vi "ex_Get Control Refnum.vi"(8 "error in (no error)":errorcluster, 9 "Name":string, 11 "Controls[]":refnum<vi>[](array[refnum])) -> (0 "error out":errorcluster, 2 "Ctl Refnum":refnum<vi>)   [LabVIEW 2020]
doc: "Returns the refnum for a control given an array of control refnums and the name of the control."
panel:
  in  "error":errorcluster={"status"=FALSE, "code"=1054, "source"="The specified object was not found."}
  out "NaN/Path/Refnum?":bool
  out "number of control refnums in":i32
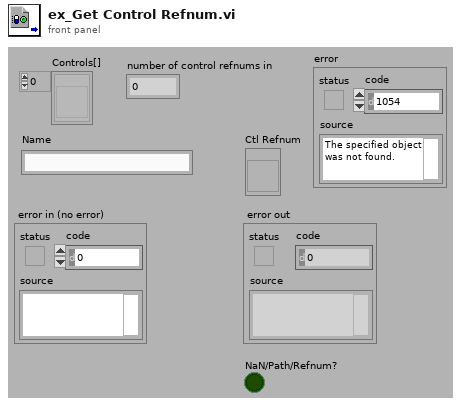
[diagram p1: front panel]
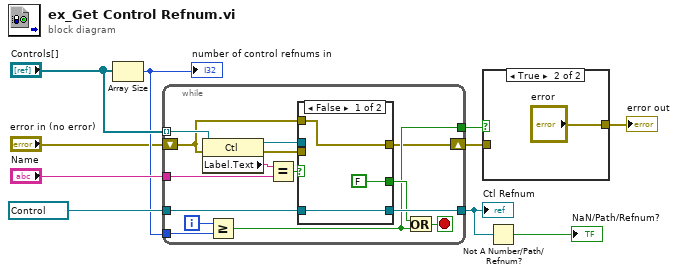
[diagram p0: block diagram]
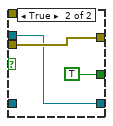
[diagram p3: hidden frame]
diagram:
  n1 = Array Size(array="Controls[]") -> (size(s)=w7:i32)
  "number of control refnums in" <- w7
  n2 = while {
    tunnel: [w25] -> w6
    tunnel: refnum<vi> refnum ("Ctl Refnum") -> [w24]
    tunnel: "Name" -> [w23]
    tunnel: "Controls[]" -> [w16] mode=indexing
    tunnel: w7 -> [w14]
    tunnel: [w13] -> w3
    shift-right: [w11] -> w1
    shift-left: "error in (no error)" -> [w12]
    i -> [w15]
    stop <- w18 stop-if-true
    n3 = property class="Ctl"(reference=w16, error in=w12) -> (reference out=w19:refnum<vi>, error out=w20:errorcluster, "Label.Text"=w21:string)
    n4 = Greater Or Equal?(x=w15, y=w14) -> (x >= y?=w13:bool)
    n5 = Equal?(x=w21, y=w23) -> (x = y?=w22:bool)
    n6 = case shown="False" w22 {
      tunnel: w20 -> [_ w31]
      tunnel: [w27 w31] -> w11
      tunnel: w19 -> [_ w30]
      tunnel: [w28 w30] -> w25
      tunnel: w24 -> [w28 _]
      tunnel: w12 -> [w27 _]
      tunnel: [FALSE TRUE] -> w17
      frame False {
      }
      frame True {
      }
    }
    n7 = Or(x=w17, y=w13) -> (x .or. y?=w18:bool)
  }
  "Ctl Refnum" <- w6
  n8 = case shown="True" w3 {
    tunnel: w1 -> [w32 _]
    tunnel: [w32 "error"] -> w4
    frame False {
    }
    frame True {
    }
  }
  "error out" <- w4
  n9 = Not A Number/Path/Refnum?(number/path/refnum=w6) -> (NaN/Path/Refnum?=→"NaN/Path/Refnum?":bool)
